vi "JSON to LVObject.vi"(8 "error in (no error)":errorcluster, 9 "JSON":string, 10 "Offset of first non-whitespace":i32, 11 "LabVIEW Object in":refnum<class>) -> (0 "error out":errorcluster, 3 "LabVIEW Object out":refnum<class>)   [LabVIEW 2019, in "JSONtext.lvlib"]
uses:
  JSONtext.lvlib
  Parsing/Advance past String.vi
  String Subset.vi
  Strip Quotes and Unescape.vi
  Unescape JSON string.vi
  Parsing/Parsing Error in converting to LabVIEW type.vi
  <vilib>/Utility/error.llb/Error Cluster From Error Code.vi
  Base64/Base64 Support.lvlib
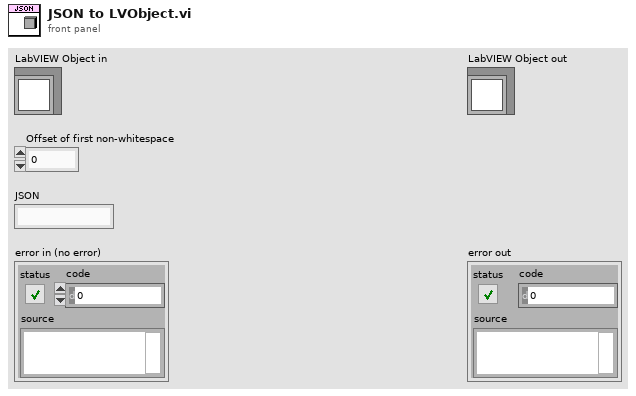
[diagram p1: front panel]
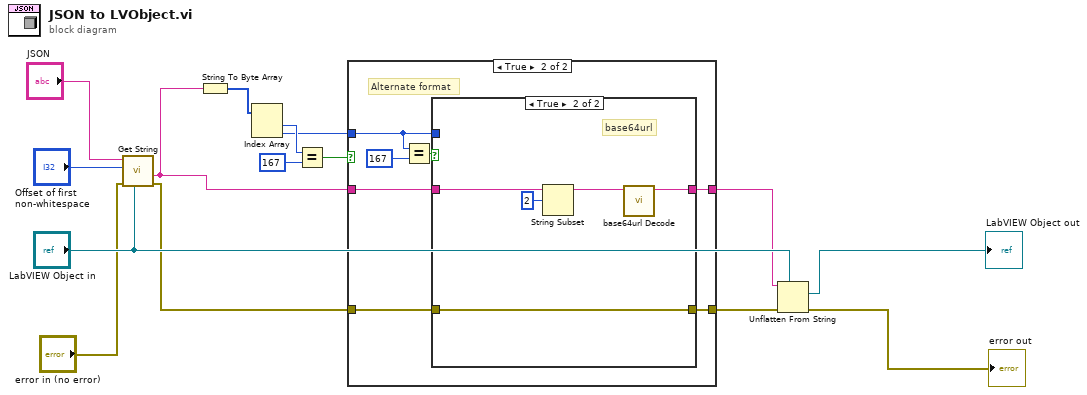
[diagram p0: block diagram]
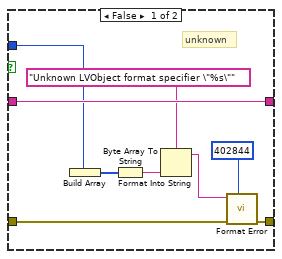
[diagram p3: hidden frame]
diagram:
  n1 = call "Get String.vi"("LV Type"="LabVIEW Object in", "error in (no error)"="error in (no error)", "Offset"="Offset of first non-whitespace", "JSON"="JSON") -> ("error out"=w1:errorcluster, "String"=w5:string)  [unwired: 5 in, 1 out]
  n2 = String To Byte Array(string=w5) -> (unsigned byte array=w10:u8[])
  n3 = Index Array(array=w10) -> (element #1=w8:u8, element #2=w6:u8)  [unwired: 2 in]
  n4 = Equal?(x=w8, y=u8 167) -> (x = y?=w7:bool)
  n5 = case shown="True" w7 {
    tunnel: w6 -> [_ w18]
    tunnel: w5 -> [w17 w23]
    tunnel: [w17 w21] -> w4
    tunnel: [w16 w19] -> w3
    tunnel: w1 -> [w16 w20]
    frame False {
    }
    frame True {
      # "Alternate format"
      n6 = Equal?(x=w18, y=u8 167) -> (x = y?=w22:bool)
      n7 = case shown="True" w22 {
        tunnel: w23 -> [w33 w38]
        tunnel: [w33 w37] -> w21
        tunnel: w20 -> [w31 w36]
        tunnel: [w32 w36] -> w19
        tunnel: w18 -> [w29 _]
        frame False {
          # "unknown"
          n8 = Build Array(w29) -> (w28:u8[])
          n9 = Byte Array To String(unsigned byte array=w28) -> (string=w27:string)
          n10 = Format Into String(format string="Unknown LVObject format specifier \"%s\"", w27) -> (resulting string=w26:string)  [unwired: 2 in, 1 out]
          n11 = call "Format Error.vi"("error code (402842)"=402844, "error in (no error)"=w31, "error message"=w26) -> ("error out"=w32:errorcluster)  [unwired: 8 in]
        }
        frame True {
          # "base64url"
          n12 = String Subset(string=w38, offset (0)=2) -> (substring=w35:string)  [unwired: 1 in]
          n13 = call "base64url Decode.vi"("Base64url (or Base64)"=w35) -> ("Decoded"=w37:string)  [unwired: 10 in]
        }
      }
    }
  }
  n14 = Unflatten From String(type="LabVIEW Object in", binary string=w4, error in (no error)=w3) -> (value=→"LabVIEW Object out":refnum<class>, error out=→"error out":errorcluster)  [unwired: 2 in, 1 out]
